vi "Log Payload.vi"(7 "Group Name":string, 8 "error in (no error)":errorcluster, 10 "tdms file":refnum<k34>, 11 "Payload in":refnum<class "Payload.lvclass">) -> (0 "error out":errorcluster, 2 "tdms file out":refnum<k34>, 3 "Payload out":refnum<class "Payload.lvclass">)   [LabVIEW 2015, in "Payload.lvclass"]
uses:
  Payload.lvclass
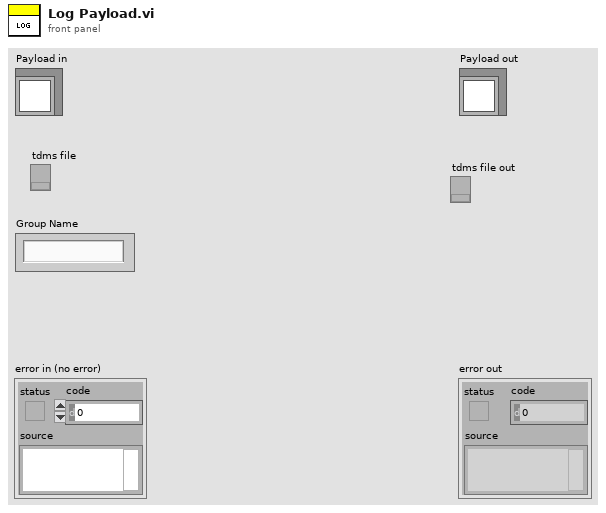
[diagram p1: front panel]
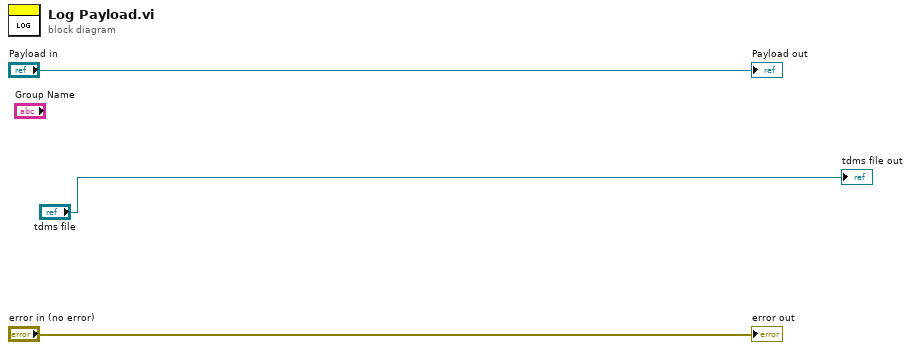
[diagram p0: block diagram]
diagram:
  "error out" <- "error in (no error)"
  "Payload out" <- "Payload in"
  "tdms file out" <- "tdms file"
